vi "DAQ.Read AI.vi"(8 "error in":errorcluster, 11 "Instrument.DAQ in":refnum<class "Instrument.DAQ.lvclass">) -> (0 "error out":errorcluster, 2 "AI []":waveform(dbl)[](array[waveform]), 3 "Instrument.DAQ out":refnum<class "Instrument.DAQ.lvclass">, 4 "AI time (ms)":u32=2)   [LabVIEW 2019, in "Instrument.DAQ.lvclass"]
uses:
  Instrument.DAQ.lvclass
  Instrument.DAQ.lvclass/Instrument.DAQ.ctl
  Typedefs/Simulation Mode--enum.ctl
  Waveguide Model/Waveguide Model--Cluster.ctl
  <vilib>/DAQmx/read.llb/DAQmx Read (Analog 1D Wfm NChan NSamp).vi
  <vilib>/DAQmx/miscellaneous.llb/DAQmx Fill In Error Info.vi
  <userlib>/_OpenG.lib/array/array.llb/Sort 1D Array (I32)__ogtk.vi
  <vilib>/Waveform/WDTOps.llb/WDT Append Waveforms DBL.vi
  <resource>/objmgr/daqmx.rc
panel:
  out "Available Samples":u32[][](graph)
  in  "show graph?":bool
  out "Ratio Chart":u32[][](graph)
  out "Waveform Graph":waveform(dbl)[](graph)
  out "P Check":bool[](array[boolean])
  out "t read (ms)":u32
  out "t check (ms)":u32
  out "Numeric":i32
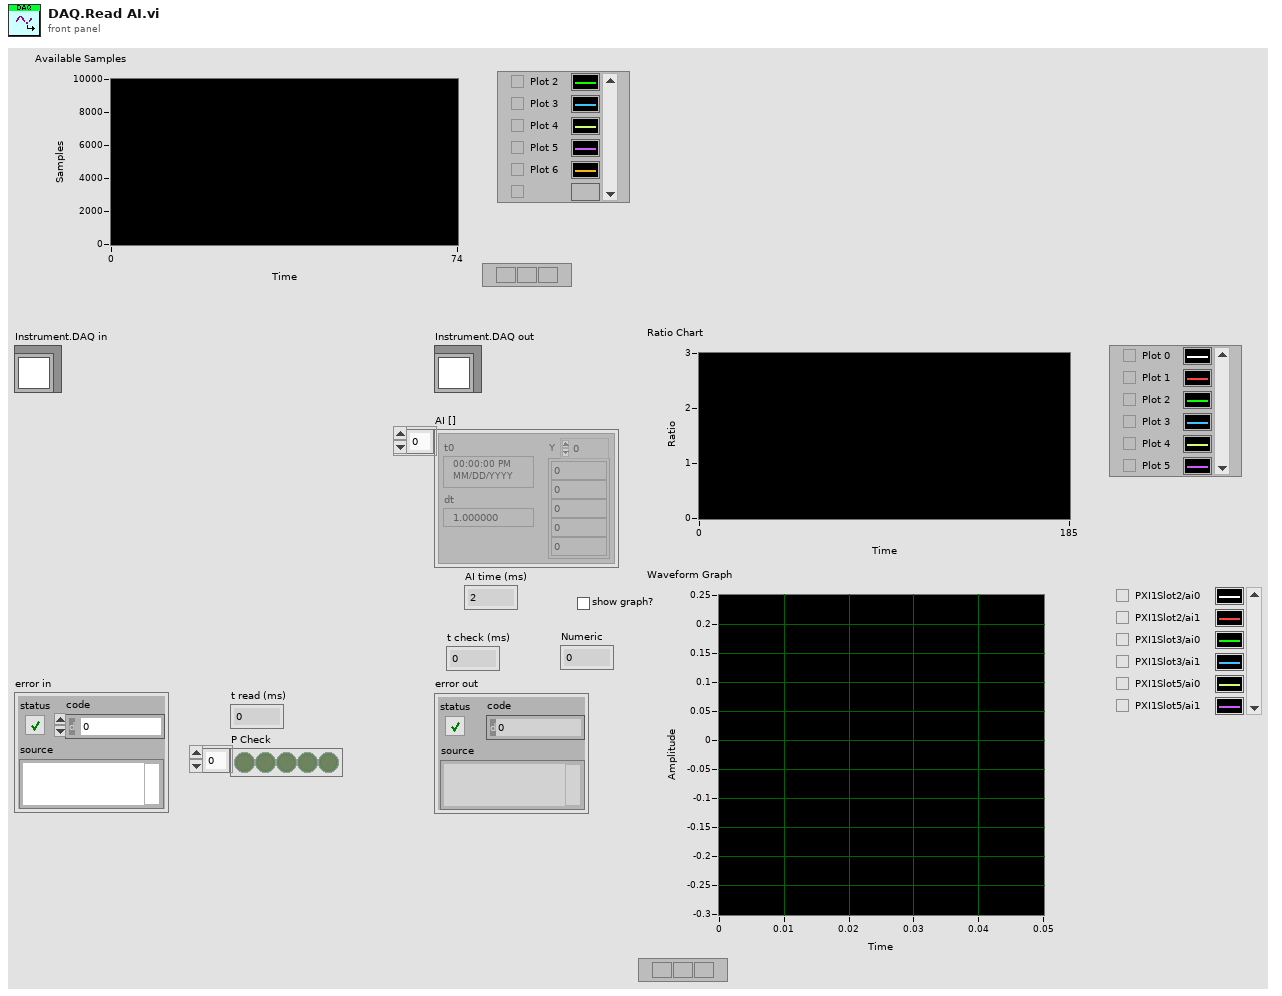
[diagram p1: front panel]
types:
  T1 = typedef "Instrument.DAQ.lvclass/Simulation Mode--enum.ctl" = enum16{"AI = HW simulated", "AI = noise*AO", "AI = waveguide"}
  T2 = typedef "Instrument.DAQ.lvclass/Waveguide Model--Cluster.ctl" = cluster{"Vsource Index":i32, "Vsg Index":i32, "V+":i32, "V-":i32}
  T3 = enum16{"static", "dynamic", "dynamic asynchronous"}
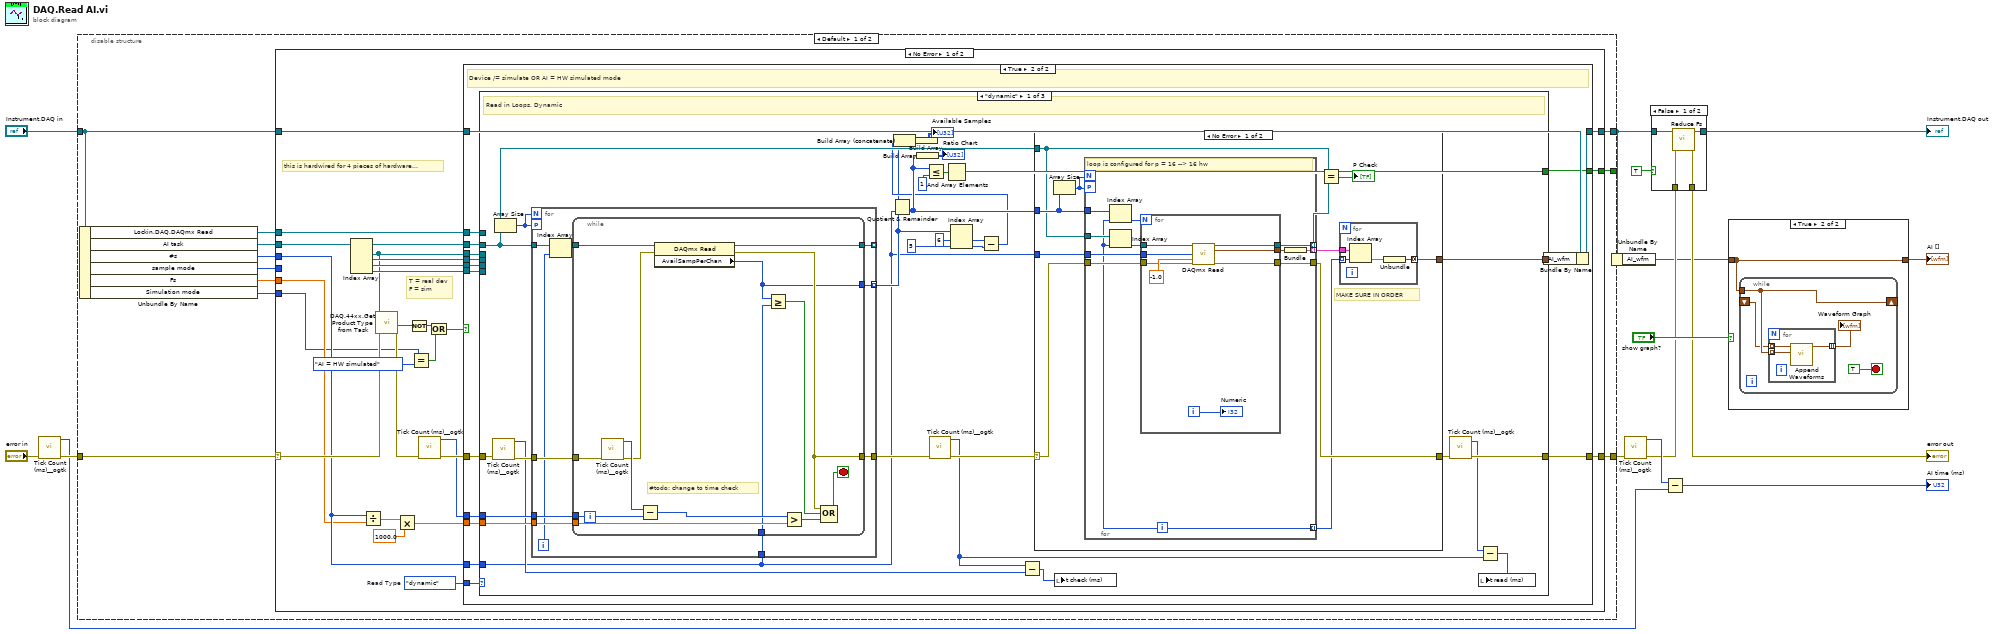
[diagram p0: block diagram]
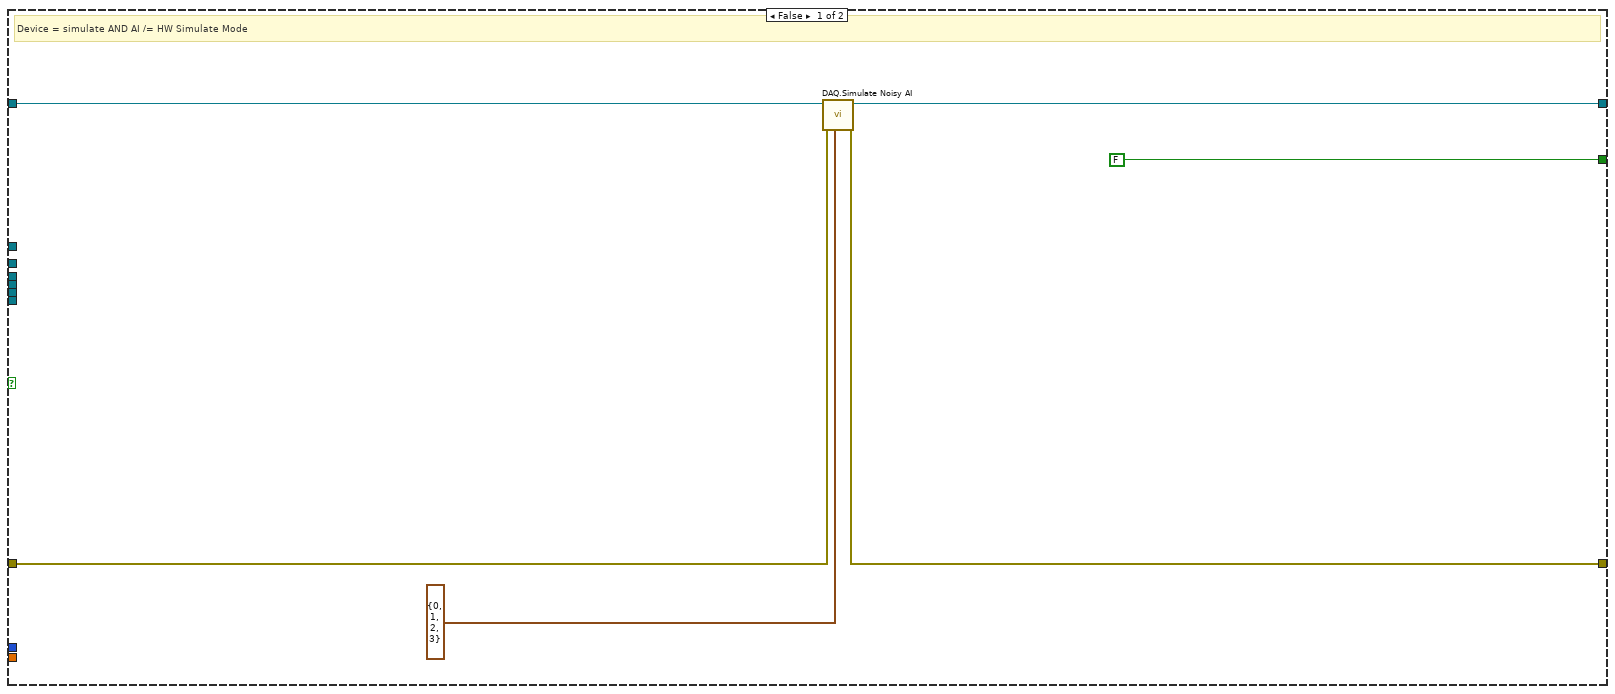
[diagram p2: hidden frame]
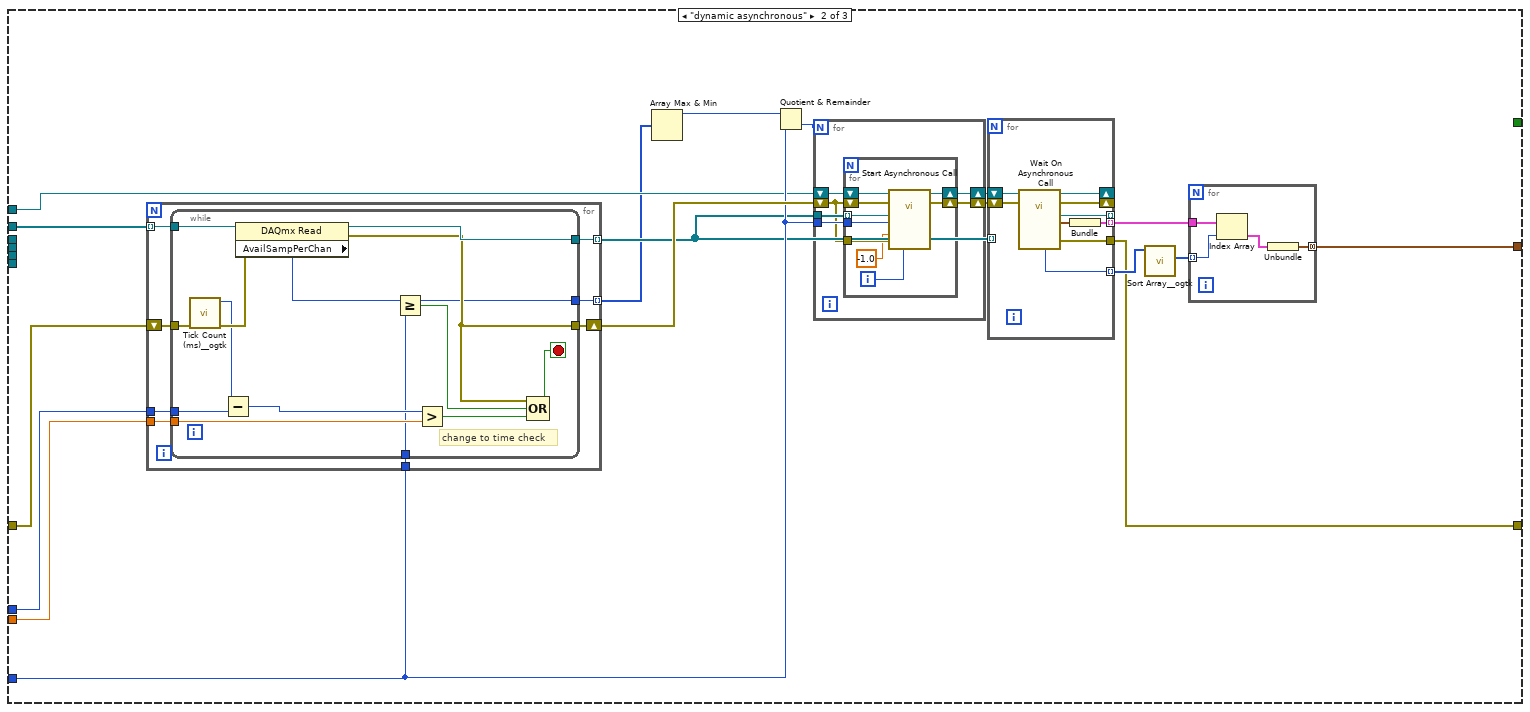
[diagram p4: hidden frame]
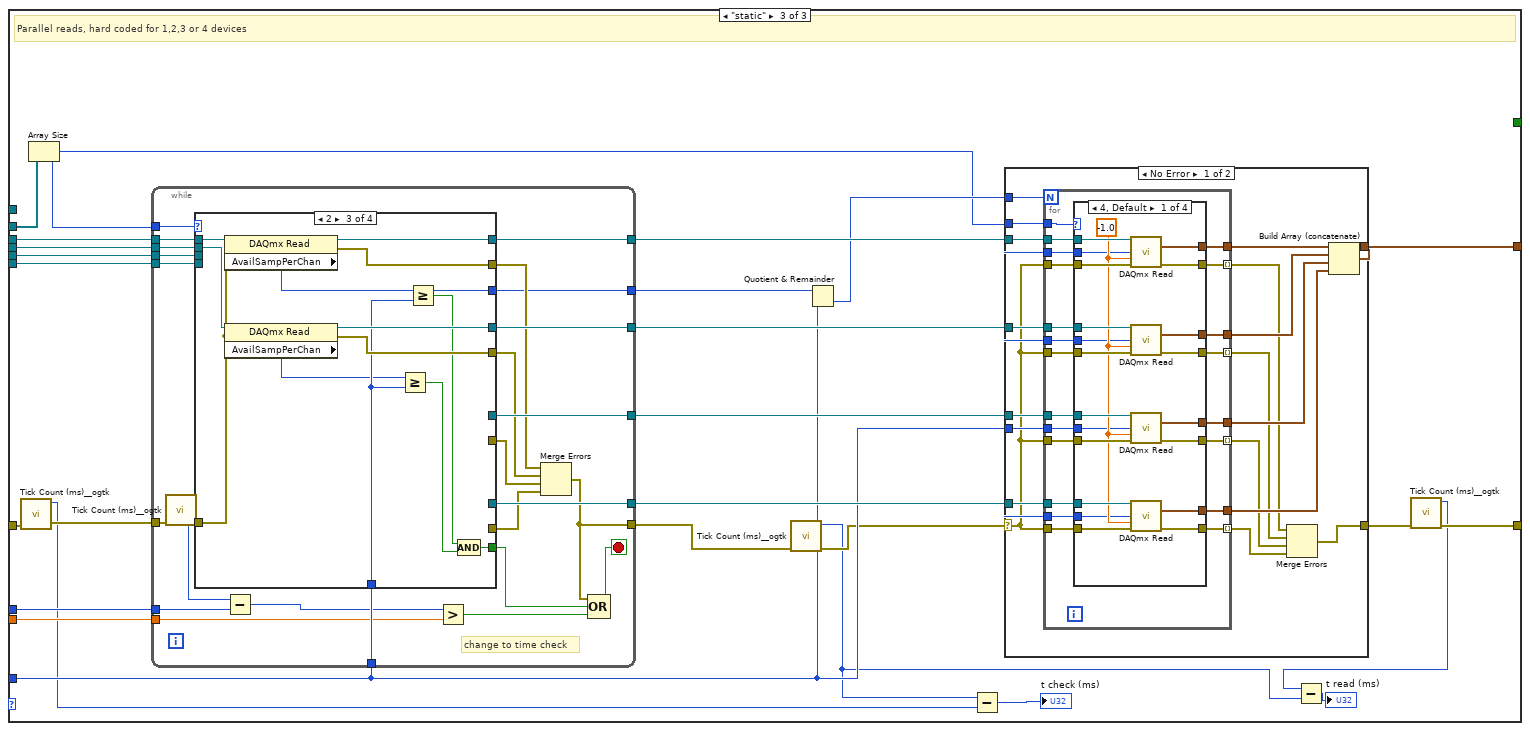
[diagram p5: hidden frame]
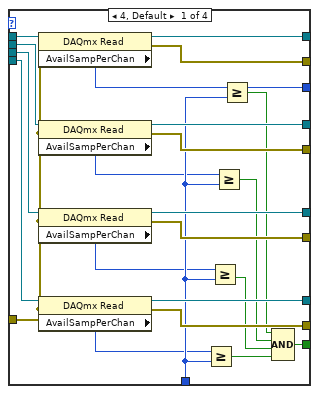
[diagram p6: hidden frame]
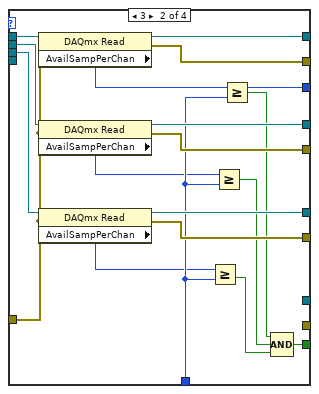
[diagram p7: hidden frame]
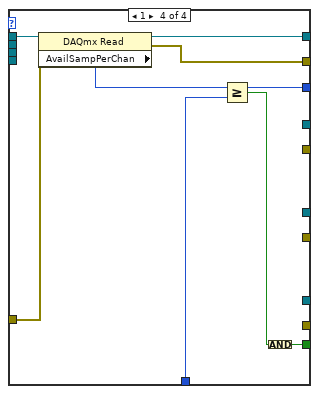
[diagram p8: hidden frame]
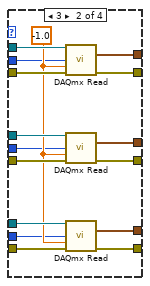
[diagram p9: hidden frame]
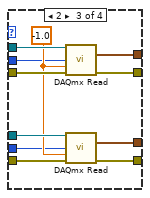
[diagram p10: hidden frame]
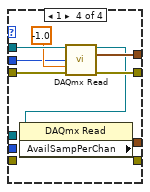
[diagram p11: hidden frame]
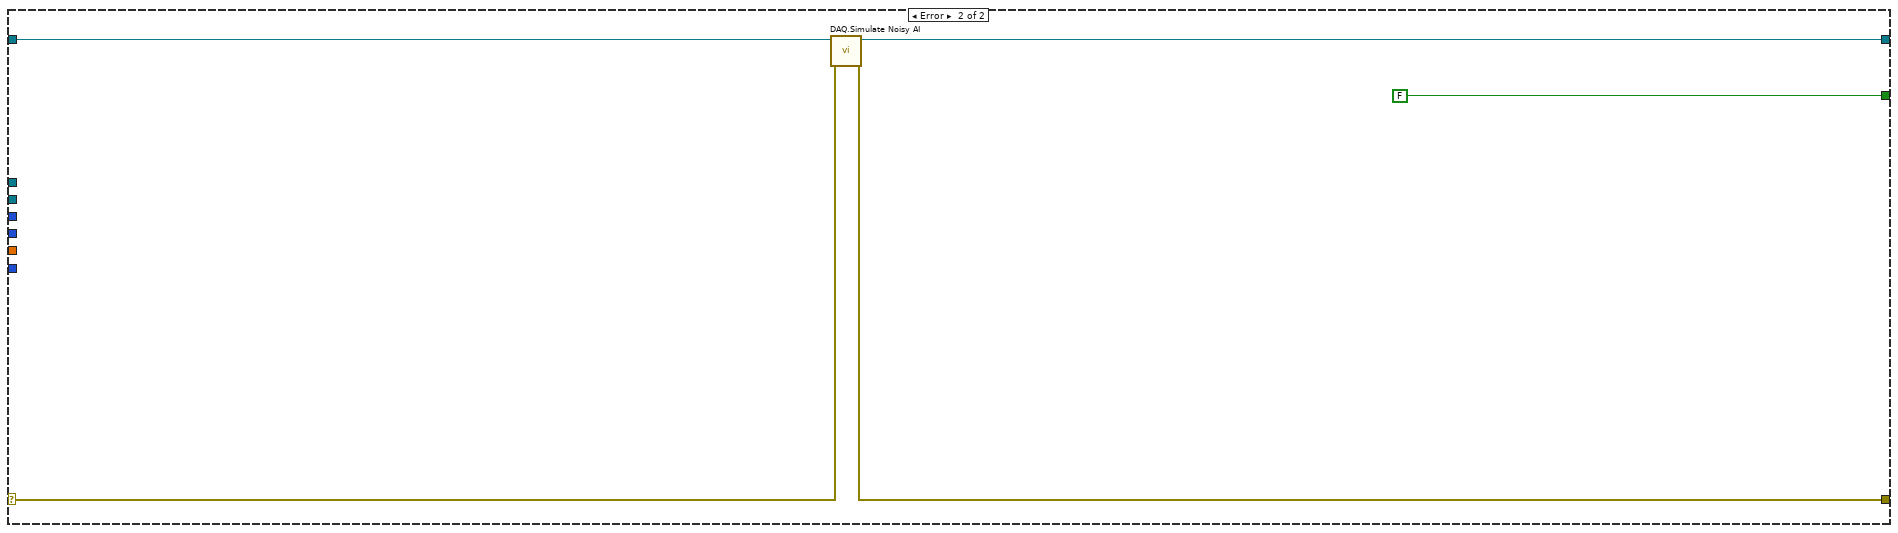
[diagram p13: hidden frame]
diagram:
  n1 = call <userlib>:"Tick Count (ms)__ogtk.vi"("error in (no error)"="error in") -> ("error out"=w14:errorcluster, "millisecond timer value"=w10:u32)  [unwired: 9 in]
  n2 = disable-structure shown="Default" {
    disable-tunnel: [w24 w447] -> w9
    disable-tunnel: "Instrument.DAQ in" -> [w23 w446]
    disable-tunnel: w14 -> [w19 w447]
    disable-tunnel: [w22 w446] -> w1
    disable-tunnel: [w16 _] -> _
    frame condition #0 (active) {
      n3 = Unbundle By Name(w23) -> ("Lockin.DAQ.DAQmx Read"=w18:refnum<vi>, "AI task"=w21:refnum<k21>[], "#s"=w26:i32, "sample mode"=w25:i32, "Fs"=w20:dbl, "Simulation mode"=w17:T1)
      n4 = case shown="No Error" w19 {
        selector: w19 -> [w46 w443]
        tunnel: w26 -> [w45 _]
        tunnel: w25 -> [_ _]
        tunnel: [w47 w444] -> w24
        tunnel: w21 -> [w37 _]
        tunnel: w23 -> [w49 w442]
        tunnel: [w29 w445] -> w22
        tunnel: w20 -> [w44 _]
        tunnel: w18 -> [w36 _]
        tunnel: w17 -> [w30 _]
        tunnel: [w27 FALSE] -> w16
        frame No Error {
          w28 = T3."dynamic"  # Read Type
          # "T = real dev\nF = sim"
          # "this is hardwired for 4 pieces of hardware..."
          n5 = Index Array(array=w37) -> (element #1=w48:refnum<k21>, element #2=w50:refnum<k21>, element #3=w51:refnum<k21>, element #4=w52:refnum<k21>)  [unwired: 4 in]
          n6 = Divide(x=w45, y=w44) -> (x/y=w43:dbl)
          n7 = call "DAQ.44xx.Get Product Type from Task.vi"("error in (no error)"=w46, "Refnum in"=w48) -> ("error out"=w40:errorcluster, "DevIsSimulated"=w33:bool)  [unwired: 6 in, 2 out]
          n8 = Multiply(x=w43, y=1000.0) -> (x*y=w39:dbl)
          n9 = Not(x=w33) -> (.not. x?=w31:bool)
          n10 = Equal?(x=w30, y=Simulation_Mode--enum."AI = HW simulated") -> (x = y?=w34:bool)
          n11 = call <userlib>:"Tick Count (ms)__ogtk.vi"("error in (no error)"=w40) -> ("error out"=w41:errorcluster, "millisecond timer value"=w38:u32)  [unwired: 9 in]
          n12 = Or(x=w31, y=w34) -> (x .or. y?=w32:bool)
          n13 = case shown="True" w32 {
            tunnel: w52 -> [_ w74]
            tunnel: w51 -> [_ w73]
            tunnel: w50 -> [_ w72]
            tunnel: w48 -> [_ w71]
            tunnel: w45 -> [_ w70]
            tunnel: w41 -> [w56 w68]
            tunnel: [w55 w69] -> w47
            tunnel: w49 -> [w58 w61]
            tunnel: w39 -> [_ w67]
            tunnel: w38 -> [_ w66]
            tunnel: w37 -> [_ w65]
            tunnel: w36 -> [_ w64]
            tunnel: [w54 w62] -> w29
            tunnel: w28 -> [_ w60]
            tunnel: [FALSE w59] -> w27
            frame False {
              # "Device = simulate AND AI /= HW Simulate Mode"
              n14 = call "DAQ.Simulate Noisy AI.vi"("Waveguide Cluster"=T2 {"Vsource Index"=0, "Vsg Index"=1, "V+"=2, "V-"=3}, "error in (no error)"=w56, "Instrument.DAQ in"=w58) -> ("error out"=w55:errorcluster, "Instrument.DAQ out"=w54:refnum<class "Instrument.DAQ.lvclass">)  [unwired: 7 in]
            }
            frame True {
              # "Device /= simulate OR AI = HW simulated mode"
              n15 = case shown="\"dynamic\"" w60 {
                tunnel: [w104 w169 w258] -> w63
                tunnel: w74 -> [_ _ w257]
                tunnel: w73 -> [_ _ w256]
                tunnel: w72 -> [_ _ w255]
                tunnel: w71 -> [_ _ w254]
                tunnel: w70 -> [w75 w173 w249]
                tunnel: [w99 w165 w239] -> w69
                tunnel: w68 -> [w101 w177 w243]
                tunnel: w67 -> [w103 w175 w248]
                tunnel: w66 -> [w102 w176 w246]
                tunnel: w65 -> [w89 w179 w234]
                tunnel: w64 -> [_ w168 _]
                tunnel: [w86 _ _] -> w59
                frame "dynamic" {
                  # "Read in Loops. Dynamic"
                  n16 = call <userlib>:"Tick Count (ms)__ogtk.vi"("error in (no error)"=w101) -> ("error out"=w100:errorcluster, "millisecond timer value"=w95:u32)  [unwired: 9 in]
                  n17 = Array Size(array=w89) -> (size(s)=w90:i32)
                  n18 = for {
                    N: w90 -> [_]
                    tunnel: w75 -> [w114]
                    tunnel: w103 -> [w112]
                    tunnel: w89 -> [w106]
                    tunnel: w102 -> [w109]
                    tunnel: [w111] -> w76 mode=indexing
                    tunnel: [w108] -> _ mode=indexing
                    workers-P: w90 -> [_]
                    tunnel: w100 -> [w113]
                    tunnel: [w110] -> w98
                    i -> [w105]
                    n19 = Index Array(array=w106, index=w105) -> (element=w107:refnum<k21>)
                    n20 = while {
                      tunnel: [w128] -> w108
                      tunnel: w113 -> [w123]
                      tunnel: [w126] -> w110
                      tunnel: w114 -> [w117]
                      tunnel: w112 -> [w124]
                      tunnel: [w118] -> w111
                      tunnel: w109 -> [w121]
                      tunnel: w107 -> [w116]
                      stop <- w127 stop-if-true
                      # "#todo: change to time check"
                      n21 = call <userlib>:"Tick Count (ms)__ogtk.vi"("error in (no error)"=w123) -> ("error out"=w115:errorcluster, "millisecond timer value"=w122:u32)  [unwired: 9 in]
                      n22 = Subtract(x=w122, y=w121) -> (x-y=w120:u32)
                      n23 = property class="DAQmx Read"(reference=w116, error in=w115) -> (reference out=w128:refnum<k21>, error out=w126:errorcluster, "AvailSampPerChan"=w118:u32)
                      n24 = Greater Or Equal?(x=w118, y=w117) -> (x >= y?=w119:bool)
                      n25 = Greater?(x=w120, y=w124) -> (0:w125:bool)
                      n26 = Compound Arithmetic op=OR(w126, w119, w125) -> (w127:bool)
                    }
                  }
                  n27 = Quotient & Remainder(x=w76, y=w75) -> (floor(x/y)=w84:u32[])  [unwired: 1 out]
                  n28 = Build Array(w84) -> (→"Ratio Chart":u32[][])
                  n29 = Less Or Equal?(x=w84, y=u32 1) -> (x <= y?=w87:bool[])
                  n30 = call <userlib>:"Tick Count (ms)__ogtk.vi"("error in (no error)"=w98) -> ("error out"=w97:errorcluster, "millisecond timer value"=w92:u32)  [unwired: 9 in]
                  n31 = And Array Elements(Boolean array=w87) -> (logical AND=w86:bool)
                  n32 = Index Array(array=w76, index #1=6 ("index"), index #2=5 ("index")) -> (element #1=w80:u32, element #2=w79:u32)
                  n33 = Subtract(x=w80, y=w79) -> (x-y=w78:u32)
                  n34 = Build Array (concatenate)(w76, w78) -> (w83:u32[])
                  n35 = Build Array(w83) -> (→"Available Samples":u32[][])
                  n36 = Subtract(x=w92, y=w95) -> (x-y=w94:u32)
                  n37 = case shown="No Error" w97 {
                    selector: w97 -> [w138 w163]
                    tunnel: [w131 _] -> w104
                    tunnel: w75 -> [w139 _]
                    tunnel: [w136 w163] -> w96
                    tunnel: w84 -> [w137 _]
                    tunnel: w89 -> [w135 _]
                    frame No Error {
                      # "MAKE SURE IN ORDER"
                      n38 = Array Size(array=w137) -> (size(s)=w129:i32)
                      n39 = for {
                        N: w129 -> [_]
                        tunnel: w139 -> [w150]
                        tunnel: [w146] -> w132 mode=indexing
                        tunnel: w137 -> [w142]
                        tunnel: w138 -> [w148]
                        tunnel: [w147] -> w136
                        tunnel: w135 -> [w143]
                        workers-P: w129 -> [_]
                        tunnel: [w141] -> w133 mode=indexing
                        tunnel: [w145] -> w130 mode=indexing
                        i -> [w141]
                        # "loop is configured for p = 16 --> 16 hw"
                        n40 = Index Array(array=w142, index=w141) -> (element=w140:u32)
                        n41 = Index Array(array=w143, index=w141) -> (element=w144:refnum<k21>)
                        n42 = for {
                          N: w140 -> [_]
                          tunnel: w144 -> [w151]
                          tunnel: w148 -> [w152]
                          tunnel: [w158] -> w149
                          tunnel: w150 -> [w153]
                          tunnel: [w157] -> w147
                          tunnel: [w154] -> w145
                          i -> [w156]
                          n43 = call-poly <vilib>:"DAQmx Read.vi"("task/channels in"=w151, "number of samples per channel"=w153, "timeout"=-1.0, "error in"=w152) -> ("task out"=w154:refnum<k21>, "data"=w158:waveform(dbl)[], "error out"=w157:errorcluster)  [unwired: 9 in]
                          "Numeric" <- w156
                        }
                        n44 = Bundle("data"=w149) -> (w146:cluster{"data":waveform(dbl)[]})  [unwired: 1 in]
                      }
                      n45 = Equal?(x=w135, y=w130) -> (x = y?=→"P Check":bool[])
                      n46 = for {
                        tunnel: w133 -> [w162] mode=indexing
                        tunnel: w132 -> [w161]
                        tunnel: [w160] -> w131 mode=concatenating
                        n47 = Index Array(array=w161, index=w162) -> (element=w159:cluster{"data":waveform(dbl)[]})
                        n48 = Unbundle(w159) -> ("data"=w160:waveform(dbl)[])
                      }
                    }
                    frame Error {
                    }
                  }
                  n49 = local write "t check (ms)"(w94) -> ()
                  n50 = call <userlib>:"Tick Count (ms)__ogtk.vi"("error in (no error)"=w96) -> ("error out"=w99:errorcluster, "millisecond timer value"=w93:u32)  [unwired: 9 in]
                  n51 = Subtract(x=w93, y=w92) -> (x-y=w91:u32)
                  n52 = local write "t read (ms)"(w91) -> ()
                }
                frame "dynamic asynchronous" {
                  n53 = for {
                    tunnel: w173 -> [w189]
                    tunnel: w175 -> [w187]
                    shift-right: [w186] -> w178
                    shift-left: w177 -> [w188]
                    tunnel: w179 -> [w184] mode=indexing
                    tunnel: w176 -> [w185]
                    tunnel: [w183] -> w172 mode=indexing
                    tunnel: [w182] -> w164 mode=indexing
                    n54 = while {
                      tunnel: [w203] -> w183
                      tunnel: w188 -> [w198]
                      tunnel: [w201] -> w186
                      tunnel: w189 -> [w191]
                      tunnel: w187 -> [w199]
                      tunnel: w185 -> [w195]
                      tunnel: w184 -> [w192]
                      tunnel: [w190] -> w182
                      stop <- w202 stop-if-true
                      # "change to time check"
                      n55 = call <userlib>:"Tick Count (ms)__ogtk.vi"("error in (no error)"=w198) -> ("error out"=w197:errorcluster, "millisecond timer value"=w196:u32)  [unwired: 9 in]
                      n56 = Subtract(x=w196, y=w195) -> (x-y=w194:u32)
                      n57 = property class="DAQmx Read"(reference=w192, error in=w197) -> (reference out=w203:refnum<k21>, error out=w201:errorcluster, "AvailSampPerChan"=w190:u32)
                      n58 = Greater Or Equal?(x=w190, y=w191) -> (x >= y?=w193:bool)
                      n59 = Greater?(x=w194, y=w199) -> (0:w200:bool)
                      n60 = Compound Arithmetic op=OR(w201, w193, w200) -> (w202:bool)
                    }
                  }
                  n61 = Array Max & Min(array=w164) -> (max value=w174:u32)  [unwired: 3 out]
                  n62 = Quotient & Remainder(x=w174, y=w173) -> (floor(x/y)=w171:u32)  [unwired: 1 out]
                  n63 = for {
                    N: w171 -> [_]
                    tunnel: w172 -> [w207]
                    tunnel: w173 -> [w205]
                    shift-right: [w208] -> w180
                    shift-left: w178 -> [w204]
                    shift-right: [w209] -> w181
                    shift-left: w168 -> [w206]
                    n64 = for {
                      shift-right: [w218] -> w208
                      shift-left: w204 -> [w215]
                      shift-right: [w217] -> w209
                      shift-left: w206 -> [w216]
                      tunnel: w204 -> [w214]
                      tunnel: w207 -> [w213] mode=indexing
                      tunnel: w205 -> [w211]
                      i -> [w210]
                      n65 = call-by-ref "Start Asynchronous Call"(reference=w216, error in=w215, "Refnum in"=w213, "number of samples per channel"=w211, "timeout"=-1.0, 11:"error in (no error)"=w214, "ID in"=w210) -> (reference out=w217:refnum<vi>, error out=w218:errorcluster)  [unwired: 7 in, 4 out]
                    }
                  }
                  n66 = for {
                    shift-right: [w224] -> _
                    shift-left: w180 -> [w226]
                    shift-right: [w225] -> _
                    shift-left: w181 -> [w227]
                    tunnel: [w221] -> _ mode=indexing
                    tunnel: [w223] -> w165
                    tunnel: [w220] -> w166 mode=indexing
                    tunnel: [w219] -> w170 mode=indexing
                    tunnel: w172 -> [_] mode=indexing
                    n67 = call-by-ref "Wait On Asynchronous Call"(reference=w227, error in=w226) -> (reference out=w225:refnum<vi>, error out=w224:errorcluster, "Refnum out"=w221:refnum<k21>, "data"=w222:waveform(dbl)[], "ID out"=w219:i32, 15:"error out"=w223:errorcluster)  [unwired: 12 in]
                    n68 = Bundle("data"=w222) -> (w220:cluster{"data":waveform(dbl)[]})  [unwired: 1 in]
                  }
                  n69 = call-poly <userlib>:"Sort Array__ogtk.vi"("Array in"=w170) -> ("Sorted Pointers"=w167:i32[])  [unwired: 9 in, 1 out]
                  n70 = for {
                    tunnel: [w231] -> w169 mode=concatenating
                    tunnel: w166 -> [w230]
                    tunnel: w167 -> [w229] mode=indexing
                    n71 = Index Array(array=w230, index=w229) -> (element=w228:cluster{"data":waveform(dbl)[]})
                    n72 = Unbundle(w228) -> ("data"=w231:waveform(dbl)[])
                  }
                }
                frame "static" {
                  # "Parallel reads, hard coded for 1,2,3 or 4 devices"
                  n73 = call <userlib>:"Tick Count (ms)__ogtk.vi"("error in (no error)"=w243) -> ("error out"=w242:errorcluster, "millisecond timer value"=w241:u32)  [unwired: 9 in]
                  n74 = Array Size(array=w234) -> (size(s)=w233:i32)
                  n75 = while {
                    tunnel: w257 -> [w283]
                    tunnel: w256 -> [w282]
                    tunnel: w255 -> [w281]
                    tunnel: w254 -> [w280]
                    tunnel: [w279] -> w253
                    tunnel: [w278] -> w252
                    tunnel: [w277] -> w251
                    tunnel: [w276] -> w250
                    tunnel: w242 -> [w264]
                    tunnel: [w265] -> w245
                    tunnel: w249 -> [w275]
                    tunnel: w233 -> [w274]
                    tunnel: w248 -> [w267]
                    tunnel: w246 -> [w261]
                    tunnel: [w259] -> w232
                    stop <- w273 stop-if-true
                    # "change to time check"
                    n76 = call <userlib>:"Tick Count (ms)__ogtk.vi"("error in (no error)"=w264) -> ("error out"=w263:errorcluster, "millisecond timer value"=w262:u32)  [unwired: 9 in]
                    n77 = case shown="2" w274 {
                      tunnel: w283 -> [w306 _ _ _]
                      tunnel: w282 -> [w305 w324 _ _]
                      tunnel: w281 -> [w304 w323 w337 _]
                      tunnel: w280 -> [w303 w322 w336 w345]
                      tunnel: [w302 w321 w335 w344] -> w279
                      tunnel: [w301 w320 w334 _] -> w278
                      tunnel: [w300 w319 _ _] -> w277
                      tunnel: [w299 _ _ _] -> w276
                      tunnel: [w298 w318 w333 w343] -> w269
                      tunnel: [w297 w317 w332 _] -> w270
                      tunnel: [w296 w316 _ _] -> w271
                      tunnel: [w295 _ _ _] -> w272
                      tunnel: w263 -> [w294 w315 w331 w342]
                      tunnel: w275 -> [w289 w311 w328 w340]
                      tunnel: [w288 w310 w327 w339] -> w266
                      tunnel: [w287 w307 w325 w338] -> w259
                      frame 4, Default {
                        n78 = property class="DAQmx Read"(reference=w303, error in=w294) -> (reference out=w302:refnum<k21>, error out=w298:errorcluster, "AvailSampPerChan"=w287:u32)
                        n79 = property class="DAQmx Read"(reference=w304, error in=w294) -> (reference out=w301:refnum<k21>, error out=w297:errorcluster, "AvailSampPerChan"=w286:u32)
                        n80 = property class="DAQmx Read"(reference=w305, error in=w294) -> (reference out=w300:refnum<k21>, error out=w296:errorcluster, "AvailSampPerChan"=w285:u32)
                        n81 = property class="DAQmx Read"(reference=w306, error in=w294) -> (reference out=w299:refnum<k21>, error out=w295:errorcluster, "AvailSampPerChan"=w284:u32)
                        n82 = Greater Or Equal?(x=w284, y=w289) -> (x >= y?=w293:bool)
                        n83 = Greater Or Equal?(x=w285, y=w289) -> (x >= y?=w292:bool)
                        n84 = Greater Or Equal?(x=w286, y=w289) -> (x >= y?=w291:bool)
                        n85 = Greater Or Equal?(x=w287, y=w289) -> (x >= y?=w290:bool)
                        n86 = Compound Arithmetic op=AND(w290, w291, w292, w293) -> (w288:bool)
                      }
                      frame 3 {
                        n87 = property class="DAQmx Read"(reference=w322, error in=w315) -> (reference out=w321:refnum<k21>, error out=w318:errorcluster, "AvailSampPerChan"=w307:u32)
                        n88 = property class="DAQmx Read"(reference=w323, error in=w315) -> (reference out=w320:refnum<k21>, error out=w317:errorcluster, "AvailSampPerChan"=w309:u32)
                        n89 = property class="DAQmx Read"(reference=w324, error in=w315) -> (reference out=w319:refnum<k21>, error out=w316:errorcluster, "AvailSampPerChan"=w308:u32)
                        n90 = Greater Or Equal?(x=w308, y=w311) -> (x >= y?=w314:bool)
                        n91 = Greater Or Equal?(x=w309, y=w311) -> (x >= y?=w313:bool)
                        n92 = Greater Or Equal?(x=w307, y=w311) -> (x >= y?=w312:bool)
                        n93 = Compound Arithmetic op=AND(w312, w313, w314) -> (w310:bool)
                      }
                      frame 2 {
                        n94 = property class="DAQmx Read"(reference=w336, error in=w331) -> (reference out=w335:refnum<k21>, error out=w333:errorcluster, "AvailSampPerChan"=w325:u32)
                        n95 = property class="DAQmx Read"(reference=w337, error in=w331) -> (reference out=w334:refnum<k21>, error out=w332:errorcluster, "AvailSampPerChan"=w326:u32)
                        n96 = Greater Or Equal?(x=w326, y=w328) -> (x >= y?=w330:bool)
                        n97 = Greater Or Equal?(x=w325, y=w328) -> (x >= y?=w329:bool)
                        n98 = Compound Arithmetic op=AND(w329, w330) -> (w327:bool)
                      }
                      frame 1 {
                        n99 = property class="DAQmx Read"(reference=w345, error in=w342) -> (reference out=w344:refnum<k21>, error out=w343:errorcluster, "AvailSampPerChan"=w338:u32)
                        n100 = Greater Or Equal?(x=w338, y=w340) -> (x >= y?=w341:bool)
                        n101 = Compound Arithmetic op=AND(w341) -> (w339:bool)
                      }
                    }
                    n102 = Subtract(x=w262, y=w261) -> (x-y=w260:u32)
                    n103 = Greater?(x=w260, y=w267) -> (0:w268:bool)
                    n104 = Merge Errors(w269, w270, w271, w272) -> (w265:errorcluster)
                    n105 = Compound Arithmetic op=OR(w265, w266, w268) -> (w273:bool)
                  }
                  n106 = call <userlib>:"Tick Count (ms)__ogtk.vi"("error in (no error)"=w245) -> ("error out"=w244:errorcluster, "millisecond timer value"=w236:u32)  [unwired: 9 in]
                  n107 = Quotient & Remainder(x=w232, y=w249) -> (floor(x/y)=w247:u32)  [unwired: 1 out]
                  n108 = Subtract(x=w236, y=w241) -> (x-y=→"t check (ms)":u32)
                  n109 = case shown="No Error" w244 {
                    selector: w244 -> [w347 w440]
                    tunnel: [w346 _] -> w258
                    tunnel: w253 -> [w363 _]
                    tunnel: w252 -> [w362 _]
                    tunnel: w251 -> [w361 _]
                    tunnel: w250 -> [w360 _]
                    tunnel: w249 -> [w356 _]
                    tunnel: [w351 w440] -> w240
                    tunnel: w233 -> [w349 _]
                    tunnel: w247 -> [w348 _]
                    frame No Error {
                      n110 = for {
                        N: w348 -> [_]
                        tunnel: w363 -> [w384]
                        tunnel: w362 -> [w383]
                        tunnel: w361 -> [w382]
                        tunnel: w360 -> [w381]
                        tunnel: w347 -> [w380]
                        tunnel: w347 -> [w379]
                        tunnel: w347 -> [w378]
                        tunnel: w347 -> [w377]
                        tunnel: [w376] -> w359
                        tunnel: [w375] -> w350
                        tunnel: [w374] -> w358
                        tunnel: [w373] -> w357
                        tunnel: w356 -> [w372]
                        tunnel: w356 -> [w371]
                        tunnel: w356 -> [w370]
                        tunnel: w356 -> [w369]
                        tunnel: [w368] -> w355 mode=indexing
                        tunnel: [w367] -> w354 mode=indexing
                        tunnel: [w366] -> w353 mode=indexing
                        tunnel: [w365] -> w352 mode=indexing
                        tunnel: w349 -> [w364]
                        n111 = case shown="4, Default" w364 {
                          tunnel: w384 -> [w405 w421 w432 w439]
                          tunnel: w383 -> [w404 w420 w431 _]
                          tunnel: w382 -> [w403 w419 _ _]
                          tunnel: w381 -> [w402 _ _ _]
                          tunnel: w380 -> [w401 w418 w430 w438]
                          tunnel: w379 -> [w400 w417 w429 _]
                          tunnel: w378 -> [w399 w416 _ _]
                          tunnel: w377 -> [w398 _ _ _]
                          tunnel: [w396 w414 w427 _] -> w376
                          tunnel: [w395 w413 w426 w436] -> w375
                          tunnel: [w394 w412 _ _] -> w374
                          tunnel: [w393 _ _ _] -> w373
                          tunnel: w372 -> [w392 _ _ _]
                          tunnel: w371 -> [w391 w411 w425 w435]
                          tunnel: w370 -> [w390 w410 _ _]
                          tunnel: w369 -> [w389 w409 w424 _]
                          tunnel: [w388 w408 w423 w434] -> w368
                          tunnel: [w387 w407 w422 _] -> w367
                          tunnel: [w386 w406 _ _] -> w366
                          tunnel: [w385 _ _ _] -> w365
                          frame 4, Default {
                            w397 = -1.0 ("timeout")
                            n112 = call-poly <vilib>:"DAQmx Read.vi"("task/channels in"=w405, "number of samples per channel"=w391, "timeout"=w397, "error in"=w401) -> ("data"=w395:waveform(dbl)[], "error out"=w388:errorcluster)  [unwired: 9 in, 1 out]
                            n113 = call-poly <vilib>:"DAQmx Read.vi"("task/channels in"=w404, "number of samples per channel"=w389, "timeout"=w397, "error in"=w400) -> ("data"=w396:waveform(dbl)[], "error out"=w387:errorcluster)  [unwired: 9 in, 1 out]
                            n114 = call-poly <vilib>:"DAQmx Read.vi"("task/channels in"=w403, "number of samples per channel"=w390, "timeout"=w397, "error in"=w399) -> ("data"=w394:waveform(dbl)[], "error out"=w386:errorcluster)  [unwired: 9 in, 1 out]
                            n115 = call-poly <vilib>:"DAQmx Read.vi"("task/channels in"=w402, "number of samples per channel"=w392, "timeout"=w397, "error in"=w398) -> ("data"=w393:waveform(dbl)[], "error out"=w385:errorcluster)  [unwired: 9 in, 1 out]
                          }
                          frame 3 {
                            w415 = -1.0 ("timeout")
                            n116 = call-poly <vilib>:"DAQmx Read.vi"("task/channels in"=w421, "number of samples per channel"=w411, "timeout"=w415, "error in"=w418) -> ("data"=w413:waveform(dbl)[], "error out"=w408:errorcluster)  [unwired: 9 in, 1 out]
                            n117 = call-poly <vilib>:"DAQmx Read.vi"("task/channels in"=w420, "number of samples per channel"=w409, "timeout"=w415, "error in"=w417) -> ("data"=w414:waveform(dbl)[], "error out"=w407:errorcluster)  [unwired: 9 in, 1 out]
                            n118 = call-poly <vilib>:"DAQmx Read.vi"("task/channels in"=w419, "number of samples per channel"=w410, "timeout"=w415, "error in"=w416) -> ("data"=w412:waveform(dbl)[], "error out"=w406:errorcluster)  [unwired: 9 in, 1 out]
                          }
                          frame 2 {
                            w428 = -1.0 ("timeout")
                            n119 = call-poly <vilib>:"DAQmx Read.vi"("task/channels in"=w432, "number of samples per channel"=w425, "timeout"=w428, "error in"=w430) -> ("data"=w426:waveform(dbl)[], "error out"=w423:errorcluster)  [unwired: 9 in, 1 out]
                            n120 = call-poly <vilib>:"DAQmx Read.vi"("task/channels in"=w431, "number of samples per channel"=w424, "timeout"=w428, "error in"=w429) -> ("data"=w427:waveform(dbl)[], "error out"=w422:errorcluster)  [unwired: 9 in, 1 out]
                          }
                          frame 1 {
                            n121 = call-poly <vilib>:"DAQmx Read.vi"("task/channels in"=w439, "number of samples per channel"=w435, "timeout"=-1.0, "error in"=w438) -> ("task out"=w433:refnum<k21>, "data"=w436:waveform(dbl)[], "error out"=w434:errorcluster)  [unwired: 9 in]
                            n122 = property class="DAQmx Read" props=["AvailSampPerChan"](reference=w433) -> ()  [unwired: 1 in, 3 out]
                          }
                        }
                      }
                      n123 = Merge Errors(w355, w354, w353, w352) -> (w351:errorcluster)
                      n124 = Build Array (concatenate)(w350, w359, w358, w357) -> (w346:waveform(dbl)[])
                    }
                    frame Error {
                    }
                  }
                  n125 = call <userlib>:"Tick Count (ms)__ogtk.vi"("error in (no error)"=w240) -> ("error out"=w239:errorcluster, "millisecond timer value"=w238:u32)  [unwired: 9 in]
                  n126 = Subtract(x=w238, y=w236) -> (x-y=→"t read (ms)":u32)
                }
              }
              n127 = Bundle By Name(cluster=w61, "AI_wfm"=w63) -> (w62:refnum<class "Instrument.DAQ.lvclass">)
            }
          }
        }
        frame Error {
          n128 = call "DAQ.Simulate Noisy AI.vi"("error in (no error)"=w443, "Instrument.DAQ in"=w442) -> ("error out"=w444:errorcluster, "Instrument.DAQ out"=w445:refnum<class "Instrument.DAQ.lvclass">)  [unwired: 8 in]
        }
      }
    }
    frame condition #1 {
    }
  }
  n129 = Unbundle By Name(w1) -> ("AI_wfm"=w4:waveform(dbl)[])
  n130 = call <userlib>:"Tick Count (ms)__ogtk.vi"("error in (no error)"=w9) -> ("error out"=w7:errorcluster, "millisecond timer value"=w13:u32)  [unwired: 9 in]
  n131 = case shown="False" TRUE {
    tunnel: w7 -> [w451 w452]
    tunnel: [w450 w452] -> w6
    tunnel: [w449 w453] -> w5
    tunnel: w1 -> [w448 w453]
    frame False {
      n132 = call "Reduce Fs.vi"("error in (no error)"=w451, "Instrument.DAQ in"=w448) -> ("error out"=w450:errorcluster, "Instrument.DAQ out"=w449:refnum<class "Instrument.DAQ.lvclass">)  [unwired: 8 in]
    }
    frame True {
    }
  }
  "error out" <- w6
  "Instrument.DAQ out" <- w5
  n133 = Subtract(x=w13, y=w10) -> (x-y=→"AI time (ms)":u32)
  n134 = case shown="True" "show graph?" {
    tunnel: w4 -> [w454 w455]
    tunnel: [w454 w455] -> w3
    frame False {
    }
    frame True {
      n135 = while {
        shift-right: [w457] -> _
        shift-left: _ -> [w456]
        tunnel: w455 -> [w457]
        stop <- TRUE stop-if-true
        n136 = for {
          tunnel: [w462] -> w458 mode=indexing
          tunnel: w456 -> [w461] mode=indexing
          tunnel: w457 -> [w460] mode=indexing
          n137 = call-poly <vilib>:"Append Waveforms.vi"("waveform B"=w460, "waveform A"=w461) -> ("waveform out"=w462:waveform(dbl))  [unwired: 8 in, 1 out]
        }
        "Waveform Graph" <- w458
      }
    }
  }
  "AI []" <- w3
